vi "TotalOffset_in_ps_Sylap.vi"(8 "error in (no error)":errorcluster, 10 "TotalOffset (ps)":dbl, 11 "VISA resource name":refnum<visa-resource-name>) -> (0 "error out":errorcluster, 2 "TotalOffset (num)":i32, 3 "VISA resource name out":refnum<visa-resource-name>)   [LabVIEW 2020]
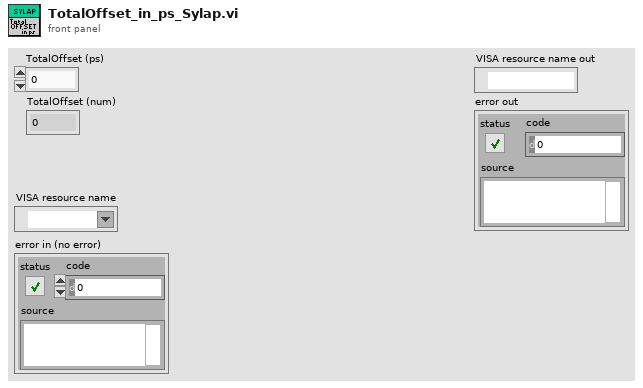
[diagram p1: front panel]
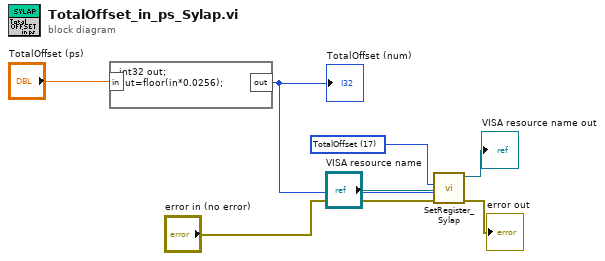
[diagram p0: block diagram]
diagram:
  w7 = u16 17 items=["Enable"=0, "TotalOffsetCoarse"=1, "PulseLength"=2, "LaserHalfLength"=3, "LaserMaxCount"=4, "TotalOffset"=17, "ResetCounters"=18, "Reset"=16] ("Register Name")
  n1 = formula code="int32 out;\nout=floor(in*0.0256);"("in"="TotalOffset (ps)") -> ("out"=w6:i32)
  "TotalOffset (num)" <- w6
  n2 = call "SetRegister_Sylap.vi"("error in (no error)"="error in (no error)", "Input Value"=w6, "Register Name"=w7, "VISA resource name"="VISA resource name") -> ("error out"=→"error out":errorcluster, "VISA resource name out"=→"VISA resource name out":refnum<visa-resource-name>)  [unwired: 4 in, 2 out]
